vi "Begin.vi"(8 "error in (no error)":errorcluster, 11 "System in":refnum<class "System.lvclass">) -> (0 "error out":errorcluster, 3 "System out":refnum<class "System.lvclass">)   [LabVIEW 2013, in "System.lvclass"]
uses:
  System.lvclass
  System.lvclass/System.ctl
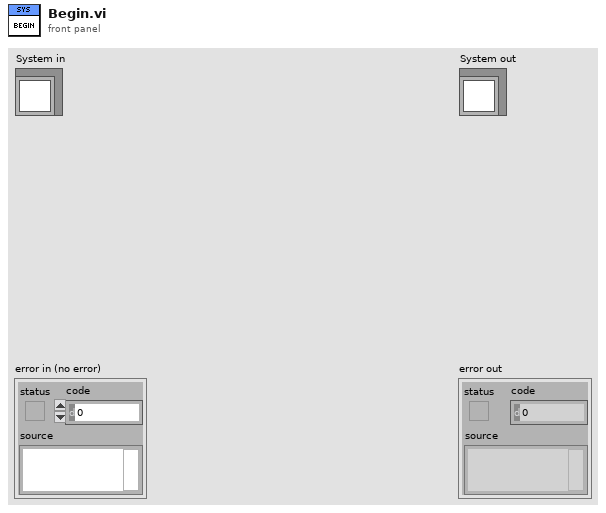
[diagram p1: front panel]
types:
  T1 = typedef "Semaphore RefNum" = refnum<k1>
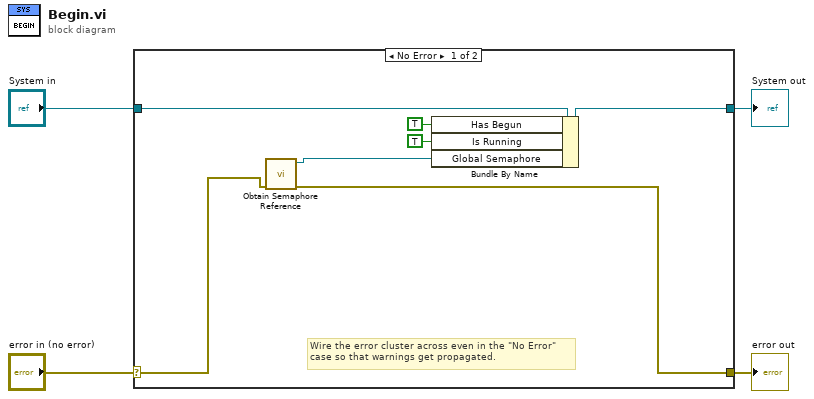
[diagram p0: block diagram]
diagram:
  n1 = case shown="No Error" "error in (no error)" {
    selector: "error in (no error)" -> [w5 w13]
    tunnel: [w6 w13] -> w3
    tunnel: [w11 w12] -> w1
    tunnel: "System in" -> [w8 w12]
    frame No Error {
      # "Wire the error cluster across even in the \"No Error\"\ncase so that warnings get propagated."
      n2 = call <vilib>:"Obtain Semaphore Reference.vi"("error in (no error)"=w5) -> ("error out"=w6:errorcluster, "semaphore"=w7:T1)  [unwired: 4 in, 1 out]
      n3 = Bundle By Name(cluster=w8, "Has Begun"=TRUE ("SystemState.Has Begun"), "Is Running"=TRUE ("SystemState.Is Running"), "Global Semaphore"=w7) -> (w11:refnum<class "System.lvclass">)
    }
    frame Error {
    }
  }
  "error out" <- w3
  "System out" <- w1
